vi "Active Power-Spectrum Method-v3_YCC.vi"() -> ()   [LabVIEW 2014]
uses:
  <vilib>/DAQmx/create/channels.llb/DAQmx Create Channel (AI-Voltage-Basic).vi
  <vilib>/DAQmx/configure/timing.llb/DAQmx Timing (Sample Clock).vi
  <vilib>/DAQmx/read.llb/DAQmx Read (Analog 1D DBL 1Chan NSamp).vi
panel:
  out "True f_drive (Hz)":dbl
  out "Real Position Array (um)":dbl[](array[numeric])
  out "Target Position Array (um)":dbl[](array[numeric])
  out "Time Array (s)":dbl[](array[numeric])
  out "QPD record time (s)":dbl
  in  "Who's Data":enum16{"YCC", "PYW", "LCH", "YYH"}(ring)
  out "All Bead Response (V)":dbl[](array[numeric])
  out "Freq. Cut for fitting":dbl[](array[numeric])
  out "best fit PSD for Thermal background":dbl[](array[numeric])
  in  "Save?":bool
  in  "Volumn of glycerol":dbl
  in  "Volumn of water":dbl=1.0
  out "A scaling":dbl
  out "True Amplitude, A (nm)":dbl
  out "Sample size per cycle":dbl
  out "df (Hz)":dbl
  in  "time per cycle (s)":dbl=0.125
  in  "Custum Fs (Hz)":i32
  in  "Sampling Rate (Hz)":T1(ring)=enum."131072"
  out "Axis":i32
  out "Real Current Commanded position (um)":dbl format="%0.5f"
  out "Sample size for all":dbl
  out "physical channels":tag
  out "stiffness from diffusion coeff.(pN/nm)":dbl
  in  "Temp (C)":dbl=25.0
  out "stiffness from friction coeff.(pN/nm)":dbl format="%#_6f"
  out "Diffusion coefficient, D (V^2/s)":dbl
  out "a1":dbl
  in  "bead height (um)":dbl=1.0
  in  "bead radius (um)":dbl=0.515
  out "Beta (V/um)":dbl
  out "fResponse (Hz)":dbl
  out "Wex":dbl
  out "Wth":dbl
  out "fc":dbl
  out "best fit parameters\n(XX,fc)":dbl[](array[numeric])
  in  "Freq End Cut":dbl=60000.0
  in  "Freq Strat Cut":dbl=50.0
  out "Frequency (Hz)\n0,df, 2df,...(n/2-1)Fs":dbl[](array[numeric])
  out "Avg. PSD":dbl[](array[numeric])
  out "Avg. completed":i32
  in  "Tab Control":enum32{"Page 1", "Time domain", "PSD"}(tab)
  out "XY Graph":T2(graph)
  out "Stage Motion":T3(graph)
  out "Bead Response Waveform":dbl[](graph)
  out "XY Graph 2":T4(graph)
  in  "Cycles to average":i32=64
  out "Sampling Rate (Hz)":i32=32000
  in  "Amplitude, A (nm)":dbl=5000.0
  in  "f_drive (Hz)":dbl=32.0
  in  "Axis (Enum)":enum16{"x", "y", "z"}(ring)
  # "fcut=80k\nfs=131072"
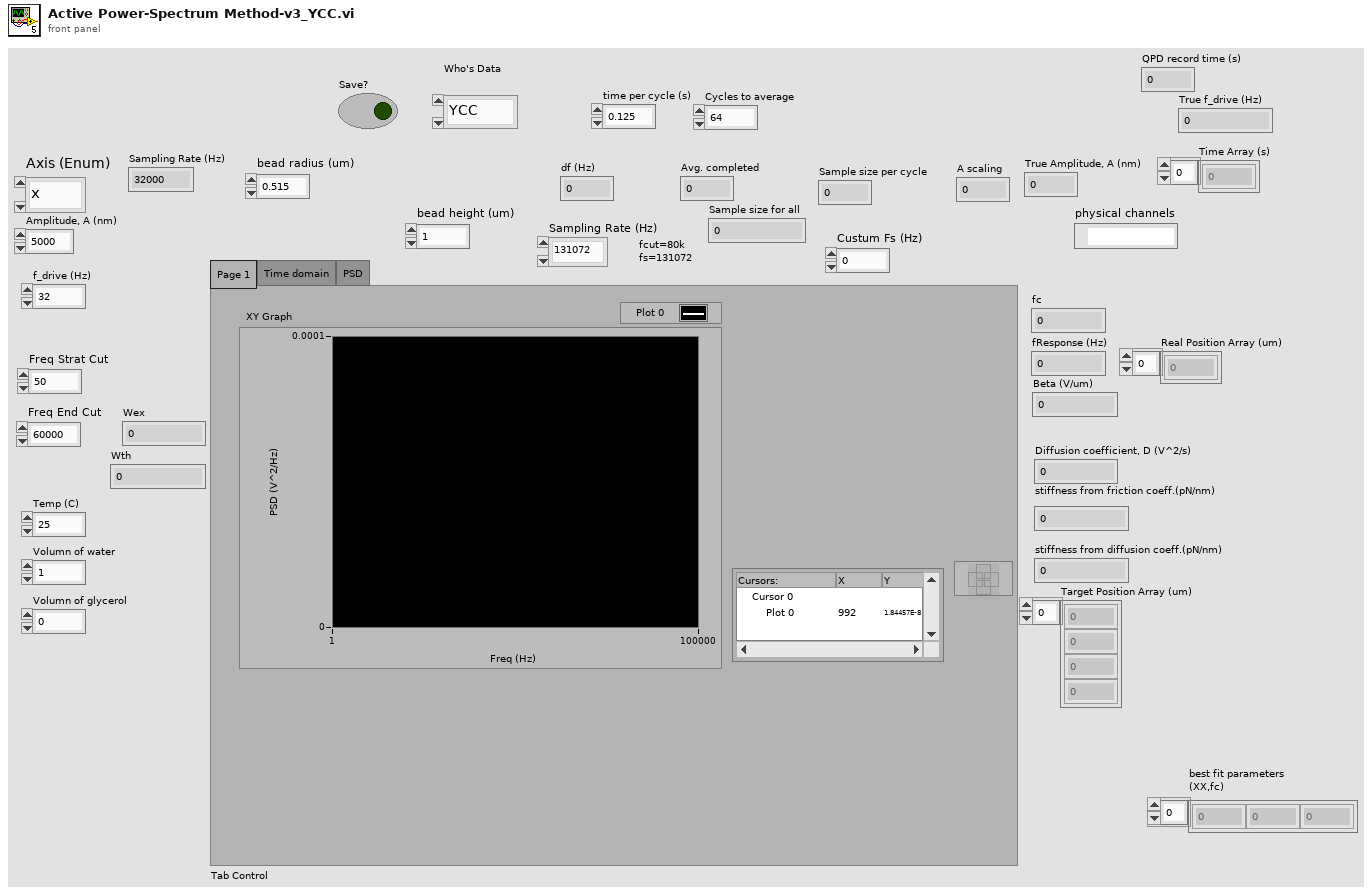
[diagram p1: front panel]
types:
  T1 = enum16{"custum", "16384", "32768", "65536", "131072", "262144"}
  T2 = cluster{"Frequency (Hz)\n0,df, 2df,...(n/2-1)Fs":dbl[], dbl[]}
  T3 = cluster{"Cut-Time Array (s)":dbl[], "best nonlinear fit for cut position":dbl[]}[]
  T4 = cluster{"Frequency (Hz)\n0,df, 2df,...(n/2-1)Fs":dbl[], dbl[]}[]
  T5 = cluster{"Cut-Time Array (s)":dbl[], "Cut-Position Array (um)":dbl[]}
  T6 = cluster{"Cut-Time Array (s)":dbl[], "best nonlinear fit for cut position":dbl[]}
  T7 = cluster{"Freq Cut":dbl[], "best nonlinear fit PSD":dbl[]}
  T8 = cluster{"Frequency (Hz)\n0,df, 2df,...(n/2-1)Fs":dbl[], "best nonlinear fit PSD":dbl[]}[]
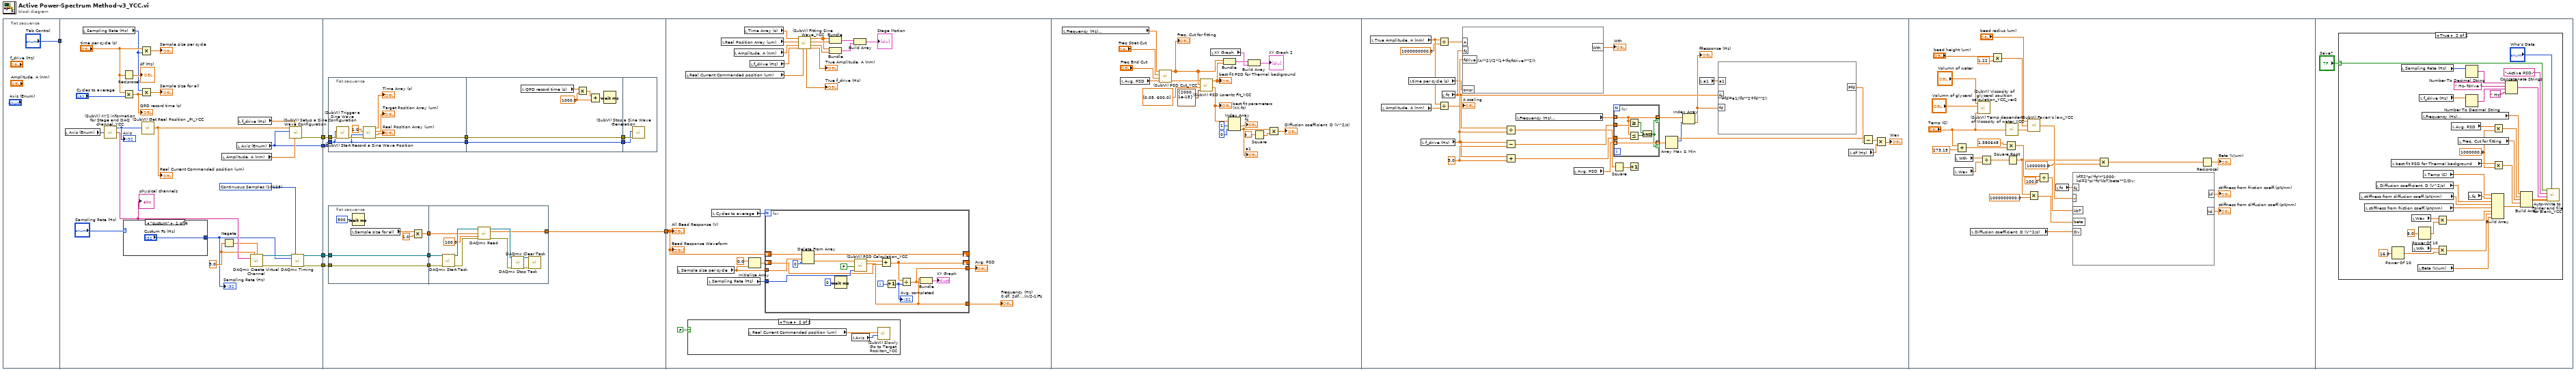
[diagram p0: block diagram]
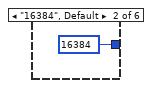
[diagram p2: hidden frame]
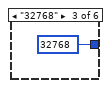
[diagram p3: hidden frame]
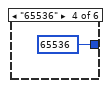
[diagram p4: hidden frame]
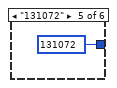
[diagram p5: hidden frame]
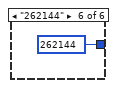
[diagram p6: hidden frame]
diagram:
  n1 = flat-sequence {
    tunnel: ["Tab Control"] -> w1
    tunnel: [w19] -> w6
    tunnel: [w18] -> w5
    tunnel: [w10] -> w3
    tunnel: [w9] -> w2
    tunnel: w1 -> [_]
    tunnel: w6 -> [w49]
    tunnel: w5 -> [w48]
    tunnel: [w47] -> w4
    tunnel: w3 -> [w43]
    tunnel: w2 -> [w42]
    tunnel: w4 -> [w102]
    frame #0 {
    }
    frame #1 {
      w26 = 10123 items=["Finite Samples"=10178, "Continuous Samples"=10123, "Hardware Timed Single Point"=12522] ("sample mode")
      w30 = 5.0 ("maximum value")
      n2 = local read "Axis (Enum)"() -> (w14:enum16{"x", "y", "z"})
      n3 = local read "Sampling Rate (Hz)"() -> (w16:i32)
      n4 = call "(SubVI) XYZ information for Stage and DAQ channel_YCC.vi"("Axis  (Enum)"=w14) -> ("physical channels"=w31:tag, "Axis"=w25:i32)  [unwired: 3 in]
      "physical channels" <- w31
      "Axis" <- w25
      n5 = Reciprocal(x="time per cycle (s)") -> (1/x=→"df (Hz)":dbl)
      n6 = Multiply(x="time per cycle (s)", y="Cycles to average") -> (x*y=w8:dbl)
      "QPD record time (s)" <- w8
      n7 = case shown="\"custum\"" "Sampling Rate (Hz)" {
        tunnel: ["Custum Fs (Hz)" 16384 32768 65536 131072 262144] -> w23
        frame "custum" {
        }
        frame "16384", Default {
        }
        frame "32768" {
        }
        frame "65536" {
        }
        frame "131072" {
        }
        frame "262144" {
        }
      }
      "Sampling Rate (Hz)" <- w23
      n8 = Multiply(x="time per cycle (s)", y=w16) -> (x*y=→"Sample size per cycle":dbl)
      n9 = Multiply(x=w16, y=w8) -> (x*y=→"Sample size for all":dbl)
      n10 = call "(SubVI) Get Real Position _PI_YCC.vi"("Axis"=w25) -> ("Real Current Commanded position (um)"=w12:dbl)  [unwired: 4 in]
      "Real Current Commanded position (um)" <- w12
      n11 = local read "Amplitude, A (nm)"() -> (w11:dbl)
      n12 = Negate(x=w30) -> (-x=w29:dbl)
      n13 = local read "Axis (Enum)"() -> (w9:enum16{"x", "y", "z"})
      n14 = local read "f_drive (Hz)"() -> (w13:dbl)
      n15 = call-poly <vilib>:"DAQmx Create Virtual Channel.vi"("maximum value"=w30, "minimum value"=w29, "physical channels"=w31) -> ("task out"=w28:refnum<k21>, "error out"=w27:errorcluster)  [unwired: 11 in]
      n16 = call "(SubVI) Setup a Sine Wave Configuration.vi"("Amplitude (nm)"=w11, "freq. (Hz)"=w13, "Axis Enum"=w9, "Current Commanded position (um)"=w12) -> ("error out"=w10:errorcluster)  [unwired: 7 in]
      n17 = call-poly <vilib>:"DAQmx Timing.vi"("task/channels in"=w28, "sample mode"=w26, "rate"=w23, "error in"=w27) -> ("task out"=w19:refnum<k21>, "error out"=w18:errorcluster)  [unwired: 3 in, 7 out]
    }
    frame #2 {
      n18 = flat-sequence {
        tunnel: w43 -> [w57]
        tunnel: w42 -> [w53]
        tunnel: [w54] -> w41
        tunnel: [w53] -> w38
        tunnel: w41 -> [w59]
        tunnel: [w59] -> w40
        tunnel: [w58] -> w39
        tunnel: w38 -> [w58]
        tunnel: w40 -> [w65]
        tunnel: w39 -> [w64]
        frame #0 {
          n19 = call "(SubVI) Trigger a Sine Wave Configuration.vi"("error in (no error)"=w57, "Axis  (Enum)"=w53) -> ("error out"=w56:errorcluster)  [unwired: 5 in]
          n20 = call "(SubVI) Start Record a Sine Wave Position.vi"("error in (no error)"=w56, "Axis (Enum)"=w53, "Record time (s)"=1.0) -> ("error out"=w54:errorcluster, "Real Position Array (um)"=→"Real Position Array (um)":dbl[], "Target Position Array (um)"=→"Target Position Array (um)":dbl[], "Time Array (s)"=→"Time Array (s)":dbl[])  [unwired: 5 in]
        }
        frame #1 {
          w61 = 1000.0 ("y")
          n21 = local read "QPD record time (s)"() -> (w63:dbl)
          n22 = Multiply(x=w63, y=w61) -> (x*y=w62:dbl)
          n23 = Add(x=w62, y=w61) -> (x+y=w60:dbl)
          n24 = Wait (ms)(milliseconds to wait=w60) -> ()  [unwired: 1 out]
        }
        frame #2 {
          n25 = call "(SubVI) Stop a Sine Wave Generation.vi"("error in (no error)"=w65, "Axis  (Enum)"=w64) -> ()  [unwired: 5 in, 1 out]
        }
      }
      n26 = flat-sequence {
        tunnel: w48 -> [w70]
        tunnel: w49 -> [w71]
        tunnel: [w71] -> w46
        tunnel: [w70] -> w45
        tunnel: [w66] -> w44
        tunnel: [w73] -> w47
        tunnel: w46 -> [w75]
        tunnel: w45 -> [w74]
        tunnel: w44 -> [w72]
        frame #0 {
          n27 = local read "Sample size for all"() -> (w67:dbl)
          n28 = Wait (ms)(milliseconds to wait=u32 500) -> ()  [unwired: 1 out]
          n29 = Multiply(x=w67, y=1.0) -> (x*y=w66:dbl)
        }
        frame #1 {
          n30 = call <vilib>:"DAQmx Start Task.vi"("task/channels in"=w75, "error in"=w74) -> ("task out"=w81:refnum<k21>, "error out"=w82:errorcluster)  [unwired: 12 out]
          n31 = call-poly <vilib>:"DAQmx Read.vi"("task/channels in"=w81, "number of samples per channel"=w72, "timeout"=100.0, "error in"=w82) -> ("task out"=w78:refnum<k21>, "data"=w73:dbl[], "error out"=w80:errorcluster)  [unwired: 9 in]
          n32 = call <vilib>:"DAQmx Stop Task.vi"("task/channels in"=w78, "error in"=w80) -> ("task out"=w76:refnum<k21>, "error out"=w77:errorcluster)  [unwired: 12 in]
          n33 = call <vilib>:"DAQmx Clear Task.vi"("task in"=w76, "error in"=w77) -> ()  [unwired: 13 in, 1 out]
        }
      }
    }
    frame #3 {
      n34 = local read "Sample size per cycle"() -> (w101:dbl)
      n35 = local read "Real Current Commanded position (um)"() -> (w91:dbl)
      n36 = case shown="True" FALSE {
        frame False {
        }
        frame True {
          n37 = local read "Real Current Commanded position (um)"() -> (w106:dbl)
          n38 = local read "Axis"() -> (w105:i32)
          n39 = call "(SubVI) Slowly Go to Target Posiiton_YCC.vi"("axis"=w105, "Target position (um)"=w106) -> ()  [unwired: 2 in, 4 out]
        }
      }
      n40 = local read "Sampling Rate (Hz)"() -> (w99:i32)
      n41 = local read "Cycles to average"() -> (w103:i32)
      n42 = local read "Real Position Array (um)"() -> (w94:dbl[])
      n43 = local read "Amplitude, A (nm)"() -> (w93:dbl)
      n44 = local read "Time Array (s)"() -> (w95:dbl[])
      n45 = Initialize Array(0.0 ("element"), w101) -> (w100:dbl[])
      n46 = local read "f_drive (Hz)"() -> (w92:dbl)
      n47 = for {
        N: w103 -> [_]
        shift-right: [w116] -> _
        shift-left: w102 -> [w119]
        tunnel: w101 -> [w118]
        shift-right: [w111] -> _
        shift-left: w100 -> [w113]
        tunnel: w99 -> [w114]
        tunnel: [w109] -> w98
        tunnel: [w108] -> w97
        i -> [w112]
        n48 = Delete From Array(array=w119, length=w118, index=0) -> (deleted portion=w115:dbl[], array with subset deleted=w116:dbl[])
        n49 = Wait (ms)(milliseconds to wait=u32 0) -> ()  [unwired: 1 out]
        n50 = call "(SubVI) PSD Calculation_YCC.vi"("sampling frequency (Hz)"=w114, "T=NI made PSD\nF=YCC made PSD"=FALSE ("T=NI made PSD\nF=YCC made PSD"), "QPD data"=w115) -> ("Frequency (Hz)\n0,df, 2df,...(n/2-1)Fs"=w109:dbl[], "Power Spectrum (V^2 rms) (V^2/Hz)"=w120:dbl[])  [unwired: 3 in]
        n51 = Add(x=w120, y=w113) -> (x+y=w111:dbl[])
        n52 = Increment(x=w112) -> (x+1=w110:i32)
        "Avg. completed" <- w110
        n53 = Divide(x=w111, y=w110) -> (x/y=w108:dbl[])
        n54 = Bundle("Frequency (Hz)\n0,df, 2df,...(n/2-1)Fs"=w109, w108) -> (→"XY Graph":T2)  [unwired: 1 in]
      }
      "Frequency (Hz)\n0,df, 2df,...(n/2-1)Fs" <- w98
      "Avg. PSD" <- w97
      n55 = call "(SubVI) Fitting Sine Wave_YCC.vi"("Start Position (um)"=w91, "f_drive (Hz)"=w92, "Amplitude, A (nm)"=w93, "Position array (um)"=w94, "Time array (s)"=w95) -> ("True Amplitude, A (nm)"=→"True Amplitude, A (nm)":dbl, "best nonlinear fit for cut position"=w88:dbl[], "Cut-Position Array (um)"=w90:dbl[], "Cut-Time Array (s)"=w89:dbl[], "True f_drive (Hz)"=→"True f_drive (Hz)":dbl)  [unwired: 1 in, 1 out]
      n56 = Bundle("Cut-Time Array (s)"=w89, "Cut-Position Array (um)"=w90) -> (w85:T5)  [unwired: 1 in]
      n57 = Bundle("Cut-Time Array (s)"=w89, "best nonlinear fit for cut position"=w88) -> (w84:T6)  [unwired: 1 in]
      n58 = Build Array(w85, w84) -> (→"Stage Motion":T3)
      "Bead Response Waveform" <- w102
      "All Bead Response (V)" <- w102
    }
    frame #4 {
      n59 = local read "Frequency (Hz)\n0,df, 2df,...(n/2-1)Fs"() -> (w126:dbl[])
      n60 = local read "Avg. PSD"() -> (w125:dbl[])
      n61 = call "(SubVI) PSD Cut_YCC.vi"("PSD"=w125, "Freq End Cut"="Freq End Cut", "Freq Strat Cut"="Freq Strat Cut", "Frequency (Hz)"=w126) -> ("PSD Cut"=w140:dbl[], "Freq Cut"=w123:dbl[])  [unwired: 2 in]
      "Freq. Cut for fitting" <- w123
      n62 = call "(SubVI) PSD Lorentz Fit_YCC.vi"("termination"=cluster{"max iteration":i32, "tolerance":dbl} {"max iteration"=2000, "tolerance"=1e-15}, "initial parameters"=dbl[] [0.05, 600.0], "Frequency (Hz)"=w123, "PSD (Vrms^2)"=w140) -> ("best fit parameters"=w134:dbl[], "best nonlinear fit PSD"=w137:dbl[])  [unwired: 2 in]
      "best fit parameters\n(XX,fc)" <- w134
      "best fit PSD for Thermal background" <- w137
      n63 = local read "XY Graph"() -> (w135:T2)
      n64 = Bundle("Freq Cut"=w123, "best nonlinear fit PSD"=w137) -> (w136:T7)  [unwired: 1 in]
      n65 = Index Array(array=w134, index #1=1 ("index"), index #2=0 ("index")) -> (element #1=→"fc":dbl, element #2=w128:dbl)
      "a1" <- w128
      n66 = Build Array(w136, w135) -> (→"XY Graph 2":T8)
      n67 = Square(x=3.141592653589793) -> (x^2=w129:dbl)
      n68 = Multiply(x=w128, y=w129) -> (x*y=→"Diffusion coefficient, D (V^2/s)":dbl)
    }
    frame #5 {
      w166 = 3.0 ("y")
      n69 = local read "True Amplitude, A (nm)"() -> (w145:dbl)
      n70 = local read "Amplitude, A (nm)"() -> (w144:dbl)
      n71 = local read "time per cycle (s)"() -> (w148:dbl)
      n72 = local read "f_drive (Hz)"() -> (w152:dbl)
      n73 = Divide(x=w145, y=1000000000.0) -> (x/y=w154:dbl)
      n74 = Divide(x=w145, y=w144) -> (x/y=→"A scaling":dbl)
      n75 = local read "fc"() -> (w153:dbl)
      n76 = formula code="Wth=(A**2)/(2*(1+(fc/fdrive)**2));"("A"=w154, "fc"=w153, "fdrive"=w152, "tmsr"=w148) -> ("Wth"=→"Wth":dbl)
      n77 = Divide(x=w153, y=w152) -> (x/y=w151:dbl)
      n78 = Subtract(x=w152, y=w166) -> (x-y=w165:dbl)
      n79 = Add(x=w152, y=w166) -> (x+y=w164:dbl)
      n80 = local read "Frequency (Hz)\n0,df, 2df,...(n/2-1)Fs"() -> (w167:dbl[])
      n81 = local read "Avg. PSD"() -> (w168:dbl[])
      n82 = Square(x=w151) -> (x^2=w150:dbl)
      n83 = for {
        tunnel: [w175] -> w163 mode=indexing if=w169
        tunnel: w168 -> [w175] mode=indexing
        tunnel: [w173] -> w162 mode=indexing if=w169
        tunnel: w167 -> [w173] mode=indexing
        tunnel: w165 -> [w174]
        tunnel: w164 -> [w172]
        n84 = Greater Or Equal?(x=w173, y=w174) -> (x >= y?=w171:bool)
        n85 = Less Or Equal?(x=w173, y=w172) -> (x <= y?=w170:bool)
        n86 = And(x=w171, y=w170) -> (x .and. y?=w169:bool)
      }
      n87 = Increment(x=w150) -> ()  [unwired: 1 out]
      n88 = Array Max & Min(array=w163) -> (max value=w159:dbl, max index (indices)=w161:i32)  [unwired: 2 out]
      n89 = Index Array(array=w162, index=w161) -> (element=w146:dbl)
      "fResponse (Hz)" <- w146
      n90 = local read "a1"() -> (w160:dbl)
      n91 = formula code="Pfd=a1/(fc**2+fd**2);"("a1"=w160, "fc"=w153, "fd"=w146) -> ("Pfd"=w147:dbl)
      n92 = local read "df (Hz)"() -> (w157:dbl)
      n93 = Subtract(x=w159, y=w147) -> (x-y=w158:dbl)
      n94 = Multiply(x=w158, y=w157) -> (x*y=→"Wex":dbl)
    }
    frame #6 {
      n95 = local read "Wex"() -> (w202:dbl)
      n96 = local read "Wth"() -> (w203:dbl)
      n97 = Add(x="Temp (C)", y=273.15) -> (x+y=w196:dbl)
      n98 = local read "Diffusion coefficient, D (V^2/s)"() -> (w189:dbl)
      n99 = call "(SubVI) Viscosity of glycerol soultion calculation_YCC_ver2.vi"("Volumn of water"="Volumn of water", "Volumn of glycerol"="Volumn of glycerol", "Temperature (C)"="Temp (C)") -> ()  [unwired: 4 in, 2 out]
      n100 = Divide(x=w203, y=w202) -> (x/y=w186:dbl)
      n101 = Multiply(x="bead height (um)", y=1.22) -> (x*y=w179:dbl)
      n102 = Multiply(x=1.380648, y=w196) -> (x*y=w195:dbl)
      n103 = call "(SubVI) Temp dependent of Viscosity of water_YCC.vi"("Temperature (C)"="Temp (C)") -> ("Viscosity (mPa*s)"=w182:dbl)  [unwired: 4 in]
      n104 = Square Root(x=w186) -> (sqrt(x)=w185:dbl)
      n105 = call "(SubVI) Faxen's law_YCC.vi"("viscosity (cP)"=w182, "bead height (um)"=w179, "bead radius (um)"="bead radius (um)") -> ("Faxen's law of friction coefficient (N/(m/s))"=w191:dbl)  [unwired: 2 in]
      n106 = Multiply(x=w185, y=1000000000.0) -> (x*y=w183:dbl)
      n107 = Divide(x=w195, y=100.0) -> (x/y=w193:dbl)
      n108 = local read "fc"() -> (w192:dbl)
      n109 = formula code="kf=2*pi*fc*r*1000;\nkd=2*pi*fc*kbT/beta**2/Dv;"("fc"=w192, "r"=w191, "kbT"=w193, "beta"=w183, "Dv"=w189) -> ("kf"=→"stiffness from friction coeff.(pN/nm)":dbl, "kd"=→"stiffness from diffusion coeff.(pN/nm)":dbl)
      n110 = Multiply(x=w185, y=1000000.0) -> (x*y=w190:dbl)
      n111 = Reciprocal(x=w190) -> (1/x=→"Beta (V/um)":dbl)
    }
    frame #7 {
      n112 = case shown="True" "Save?" {
        selector: "Save?" -> [_ w237]
        frame False {
        }
        frame True {
          w215 = 1000000.0 ("y")
          n113 = local read "stiffness from diffusion coeff.(pN/nm)"() -> (w231:dbl)
          n114 = local read "stiffness from friction coeff.(pN/nm)"() -> (w230:dbl)
          n115 = local read "Diffusion coefficient, D (V^2/s)"() -> (w232:dbl)
          n116 = local read "best fit PSD for Thermal background"() -> (w216:dbl[])
          n117 = Power Of 10(x=16.0) -> (10^x=w212:dbl)
          n118 = local read "Sampling Rate (Hz)"() -> (w225:i32)
          n119 = local read "Wex"() -> (w208:dbl)
          n120 = local read "Wth"() -> (w206:dbl)
          n121 = local read "Beta (V/um)"() -> (w213:dbl)
          n122 = Power Of 10(x=6.0) -> (10^x=w209:dbl)
          n123 = local read "f_drive (Hz)"() -> (w222:dbl)
          n124 = local read "Frequency (Hz)\n0,df, 2df,...(n/2-1)Fs"() -> (w235:dbl[])
          n125 = local read "Temp (C)"() -> (w226:dbl)
          n126 = Multiply(x=w208, y=w209) -> (x*y=w207:dbl)
          n127 = Multiply(x=w206, y=w212) -> (x*y=w205:dbl)
          n128 = local read "Avg. PSD"() -> (w218:dbl[])
          n129 = local read "Freq. Cut for fitting"() -> (w234:dbl[])
          n130 = Number To Decimal String(number=w225) -> (decimal integer string=w224:string)  [unwired: 1 in]
          n131 = Number To Decimal String(number=w222) -> (decimal integer string=w221:string)  [unwired: 1 in]
          n132 = local read "fc"() -> (w233:dbl)
          n133 = Build Array(w226, w233, w232, w231, w230, w207, w205, w213) -> (w229:dbl[])
          n134 = Multiply(x=w218, y=w215) -> (x*y=w217:dbl[])
          n135 = Multiply(x=w216, y=w215) -> (x*y=w214:dbl[])
          n136 = Concatenate Strings(w224, " Hz- fdrive " ("string"), w221, " Hz" ("string")) -> (w219:string)
          n137 = Build Array(w235, w217, w234, w214, w229) -> (w228:dbl[][])
          n138 = call "Auto-Write to Folder and file for Blank_YCC.vi"("Who's Data"="Who's Data", "data to be saved"=w228, "File name add to the end \n(height)"=w219, "Title"="-Active PSD-", "Save?"=w237) -> ()  [unwired: 3 in, 2 out]
        }
      }
    }
  }
